vi "ErrorCycleNoSet.vi"(8 "error in":errorcluster, 10 "CaseNo":enum16{"S2", "S3", "S4", "S11"}(ring), 11 "Error Set Item":string="$AlarmCycleNo_S2") -> (0 "error out":errorcluster)   [LabVIEW 2019]
uses:
  Global/Process Global.vi
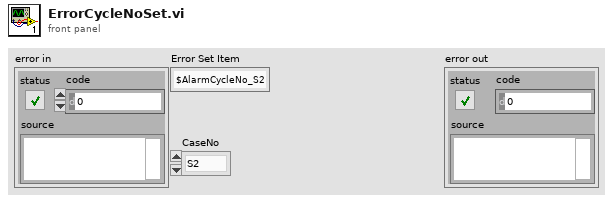
[diagram p1: front panel]
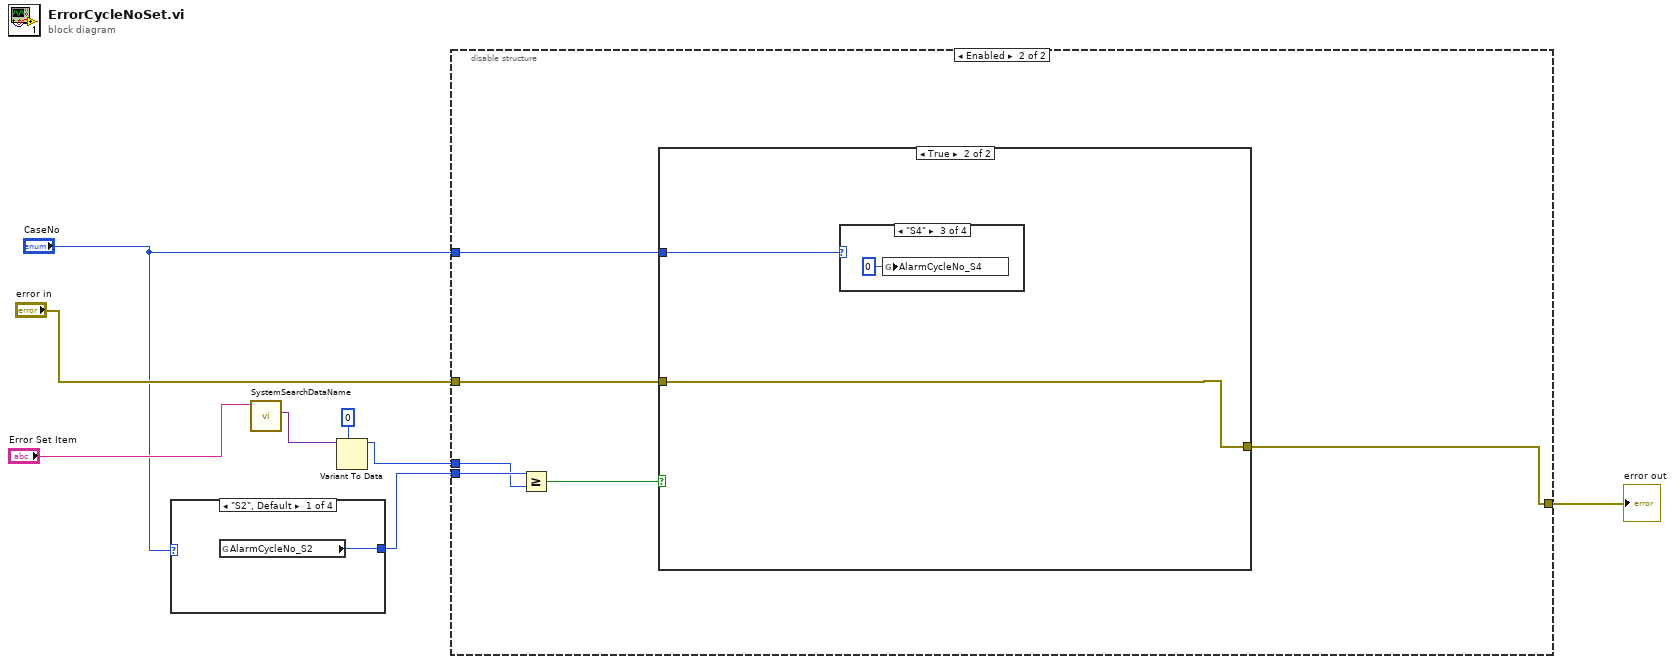
[diagram p0: block diagram]
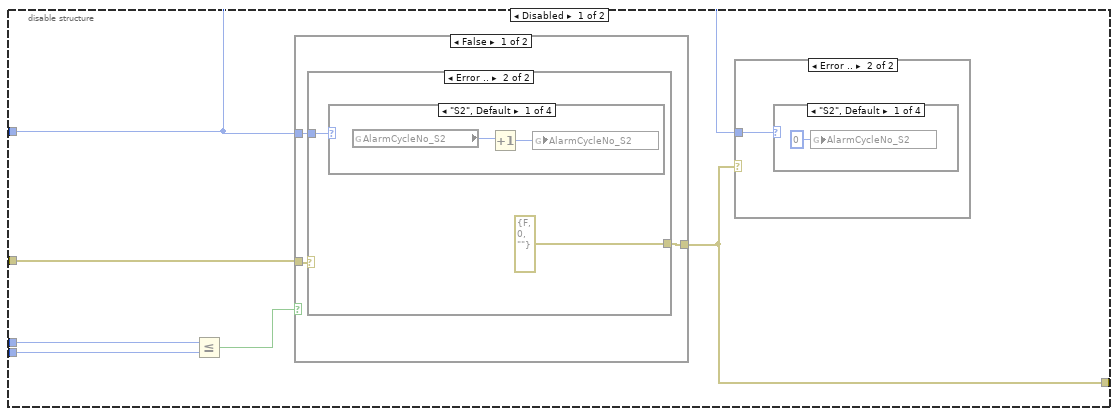
[diagram p2: hidden frame]
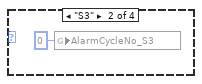
[diagram p4: hidden frame]
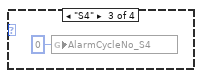
[diagram p5: hidden frame]
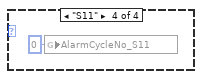
[diagram p6: hidden frame]
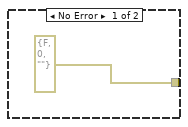
[diagram p7: hidden frame]
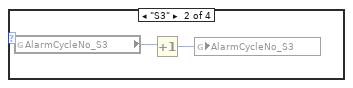
[diagram p8: hidden frame]
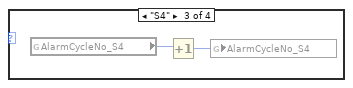
[diagram p9: hidden frame]
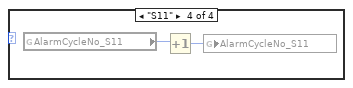
[diagram p10: hidden frame]
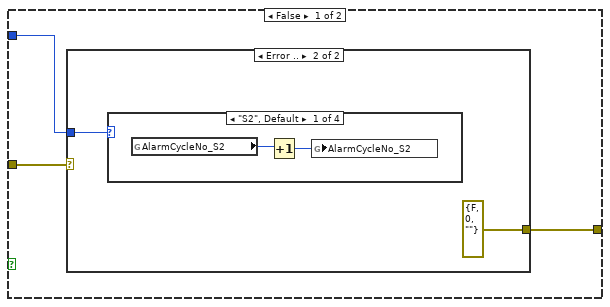
[diagram p12: hidden frame]
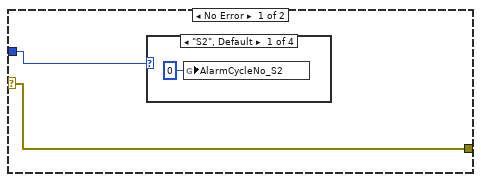
[diagram p13: hidden frame]
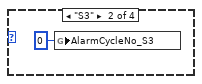
[diagram p14: hidden frame]
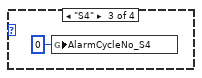
[diagram p15: hidden frame]
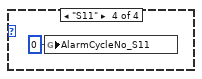
[diagram p16: hidden frame]
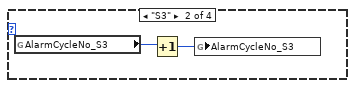
[diagram p17: hidden frame]
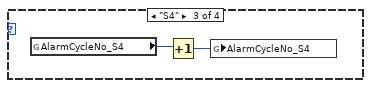
[diagram p18: hidden frame]
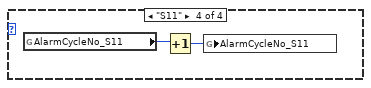
[diagram p19: hidden frame]
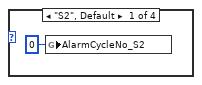
[diagram p20: hidden frame]
diagram:
  n1 = case shown="\"S2\", Default" "CaseNo" {
    tunnel: [w9 w10 w11 w12] -> w1
    frame "S2", Default {
      n2 = global read "Process Global.vi" "AlarmCycleNo_S2"() -> (w9:i16)
    }
    frame "S3" {
      n3 = global read "Process Global.vi" "AlarmCycleNo_S3"() -> (w10:i16)
    }
    frame "S4" {
      n4 = global read "Process Global.vi" "AlarmCycleNo_S4"() -> (w11:i16)
    }
    frame "S11" {
      n5 = global read "Process Global.vi" "AlarmCycleNo_S11"() -> (w12:i16)
    }
  }
  n6 = call "SystemSearchDataName.vi"("element"="Error Set Item") -> ("variant"=w5:variant)  [unwired: 8 in, 2 out]
  n7 = Variant To Data(type=i16 0 ("Numeric"), Variant=w5) -> (data=w7:i16)  [unwired: 1 in, 1 out]
  n8 = disable-structure shown="Enabled" {
    disable-tunnel: [w18 w39] -> w8
    disable-tunnel: w7 -> [w16 w43]
    disable-tunnel: "error in" -> [w15 w41]
    disable-tunnel: "CaseNo" -> [w14 w40]
    disable-tunnel: w1 -> [w13 w44]
    frame Disabled {
      n9 = Less Or Equal?(x=w16, y=w13) -> (x <= y?=w17:bool)
      n10 = case shown="False" w17 {
        tunnel: w15 -> [w25 w38]
        tunnel: [w26 w38] -> w18
        tunnel: w14 -> [w24 _]
        frame False {
          n11 = case shown="Error .." w25 {
            tunnel: [errorcluster {"status"=FALSE, "code"=0, "source"=""} ("error IO") errorcluster {"status"=FALSE, "code"=0, "source"=""} ("error IO")] -> w26
            tunnel: w24 -> [_ w28]
            frame No Error {
            }
            frame Error {
              n12 = case shown="\"S2\", Default" w28 {
                frame "S2", Default {
                  n13 = global read "Process Global.vi" "AlarmCycleNo_S2"() -> (w31:i16)
                  n14 = Increment(x=w31) -> (x+1=w30:i16)
                  n15 = global write "Process Global.vi" "AlarmCycleNo_S2"(w30) -> ()
                }
                frame "S3" {
                  n16 = global read "Process Global.vi" "AlarmCycleNo_S3"() -> (w33:i16)
                  n17 = Increment(x=w33) -> (x+1=w32:i16)
                  n18 = global write "Process Global.vi" "AlarmCycleNo_S3"(w32) -> ()
                }
                frame "S4" {
                  n19 = global read "Process Global.vi" "AlarmCycleNo_S4"() -> (w35:i16)
                  n20 = Increment(x=w35) -> (x+1=w34:i16)
                  n21 = global write "Process Global.vi" "AlarmCycleNo_S4"(w34) -> ()
                }
                frame "S11" {
                  n22 = global read "Process Global.vi" "AlarmCycleNo_S11"() -> (w37:i16)
                  n23 = Increment(x=w37) -> (x+1=w36:i16)
                  n24 = global write "Process Global.vi" "AlarmCycleNo_S11"(w36) -> ()
                }
              }
            }
          }
        }
        frame True {
        }
      }
      n25 = case shown="Error .." w18 {
        tunnel: w14 -> [_ w19]
        frame No Error {
        }
        frame Error {
          n26 = case shown="\"S2\", Default" w19 {
            frame "S2", Default {
              n27 = global write "Process Global.vi" "AlarmCycleNo_S2"(i16 0 ("AlarmCycleNo")) -> ()
            }
            frame "S3" {
              n28 = global write "Process Global.vi" "AlarmCycleNo_S3"(i16 0 ("AlarmCycleNo")) -> ()
            }
            frame "S4" {
              n29 = global write "Process Global.vi" "AlarmCycleNo_S4"(i16 0 ("AlarmCycleNo")) -> ()
            }
            frame "S11" {
              n30 = global write "Process Global.vi" "AlarmCycleNo_S11"(i16 0 ("AlarmCycleNo")) -> ()
            }
          }
        }
      }
    }
    frame Enabled {
      n31 = Greater Or Equal?(x=w44, y=w43) -> (x >= y?=w42:bool)
      n32 = case shown="True" w42 {
        tunnel: w41 -> [w47 w65]
        tunnel: w40 -> [w46 w64]
        tunnel: [w45 w65] -> w39
        frame False {
          n33 = case shown="Error .." w47 {
            selector: w47 -> [w48 _]
            tunnel: w46 -> [w49 w55]
            tunnel: [w48 errorcluster {"status"=FALSE, "code"=0, "source"=""} ("error out")] -> w45
            frame No Error {
              n34 = case shown="\"S2\", Default" w49 {
                frame "S2", Default {
                  n35 = global write "Process Global.vi" "AlarmCycleNo_S2"(i16 0 ("AlarmCycleNo")) -> ()
                }
                frame "S3" {
                  n36 = global write "Process Global.vi" "AlarmCycleNo_S3"(i16 0 ("AlarmCycleNo")) -> ()
                }
                frame "S4" {
                  n37 = global write "Process Global.vi" "AlarmCycleNo_S4"(i16 0 ("AlarmCycleNo")) -> ()
                }
                frame "S11" {
                  n38 = global write "Process Global.vi" "AlarmCycleNo_S11"(i16 0 ("AlarmCycleNo")) -> ()
                }
              }
            }
            frame Error {
              n39 = case shown="\"S2\", Default" w55 {
                frame "S2", Default {
                  n40 = global read "Process Global.vi" "AlarmCycleNo_S2"() -> (w57:i16)
                  n41 = Increment(x=w57) -> (x+1=w56:i16)
                  n42 = global write "Process Global.vi" "AlarmCycleNo_S2"(w56) -> ()
                }
                frame "S3" {
                  n43 = global read "Process Global.vi" "AlarmCycleNo_S3"() -> (w59:i16)
                  n44 = Increment(x=w59) -> (x+1=w58:i16)
                  n45 = global write "Process Global.vi" "AlarmCycleNo_S3"(w58) -> ()
                }
                frame "S4" {
                  n46 = global read "Process Global.vi" "AlarmCycleNo_S4"() -> (w61:i16)
                  n47 = Increment(x=w61) -> (x+1=w60:i16)
                  n48 = global write "Process Global.vi" "AlarmCycleNo_S4"(w60) -> ()
                }
                frame "S11" {
                  n49 = global read "Process Global.vi" "AlarmCycleNo_S11"() -> (w63:i16)
                  n50 = Increment(x=w63) -> (x+1=w62:i16)
                  n51 = global write "Process Global.vi" "AlarmCycleNo_S11"(w62) -> ()
                }
              }
            }
          }
        }
        frame True {
          n52 = case shown="\"S4\"" w64 {
            frame "S2", Default {
              n53 = global write "Process Global.vi" "AlarmCycleNo_S2"(i16 0 ("AlarmCycleNo")) -> ()
            }
            frame "S3" {
              n54 = global write "Process Global.vi" "AlarmCycleNo_S3"(i16 0 ("AlarmCycleNo")) -> ()
            }
            frame "S4" {
              n55 = global write "Process Global.vi" "AlarmCycleNo_S4"(i16 0 ("AlarmCycleNo")) -> ()
            }
            frame "S11" {
              n56 = global write "Process Global.vi" "AlarmCycleNo_S11"(i16 0 ("AlarmCycleNo")) -> ()
            }
          }
        }
      }
    }
  }
  "error out" <- w8
